vi "Parameters.vi"(8 "error in (no error)":errorcluster, 11 "Temperature Converter Test In":refnum<class "Temperature Converter Test.lvclass">) -> (0 "error out":errorcluster, 2 "Parameters":T1(array[cluster]))   [LabVIEW 2020, in "Temperature Converter Test.lvclass"]
uses:
  Temperature Converter Test.lvclass
  C:/git/astemes-lunit-parameterized-test/source/Parameterized Test Case/Parameterized Test Case.lvclass
  source/Parameterized Test Case/Parameterized Test Case.lvclass
  Temperature Converter Test.lvclass/Temperature Converter Test.ctl
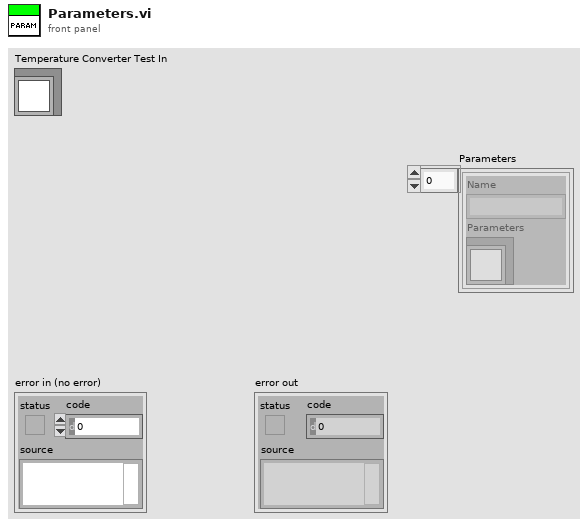
[diagram p1: front panel]
types:
  T1 = cluster{"Name":string, "Parameters":refnum<class "Parameterized Test Case.lvclass">}[]
  T2 = cluster{"In":dbl, "Direction":enum16{"F to C", "C to F"}, "Expected Out":dbl}[]
  T3 = cluster{string, "Temperature Converter Test.lvclass":refnum<class "Temperature Converter Test.lvclass">}
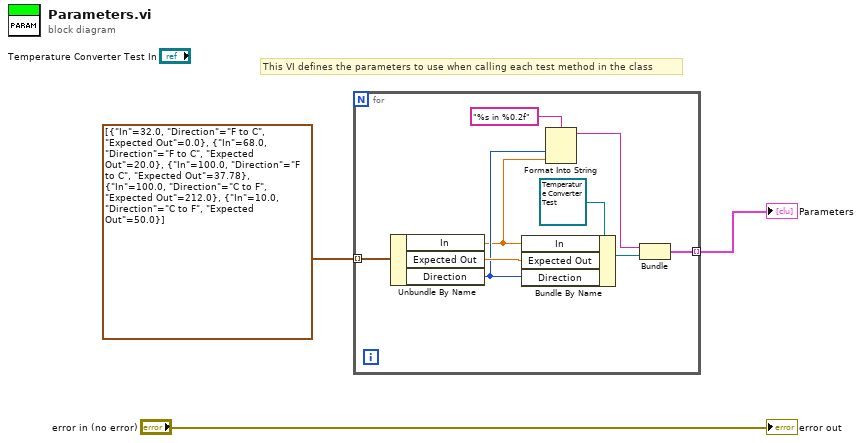
[diagram p0: block diagram]
diagram:
  # "This VI defines the parameters to use when calling each test method in the class"
  n1 = for {
    tunnel: [w9] -> w2 mode=indexing
    tunnel: T2 [{"In"=32.0, "Direction"=enum."F to C", "Expected Out"=0.0}, {"In"=68.0, "Direction"=enum."F to C", "Expected Out"=20.0}, {"In"=100.0, "Direction"=enum."F to C", "Expected Out"=37.78}, {"In"=100.0, "Direction"=enum."C to F", "Expected Out"=212.0}, {"In"=10.0, "Direction"=enum."C to F", "Expected Out"=50.0}] -> [w7] mode=indexing
    n2 = Unbundle By Name(w7) -> ("In"=w4:dbl, "Expected Out"=w6:dbl, "Direction"=w5:enum16{"F to C", "C to F"})
    n3 = Bundle By Name(cluster=refnum<class "Temperature Converter Test.lvclass"> refnum ("Temperature Converter Test.lvclass"), "In"=w4, "Expected Out"=w6, "Direction"=w5) -> (w11:refnum<class "Temperature Converter Test.lvclass">)
    n4 = Format Into String(format string="%s in %0.2f", w5, w4) -> (resulting string=w10:string)  [unwired: 2 in, 1 out]
    n5 = Bundle(w10, "Temperature Converter Test.lvclass"=w11) -> (w9:T3)  [unwired: 1 in]
  }
  "Parameters" <- w2
  "error out" <- "error in (no error)"
